vi "Delete SIM Profile.vi"(8 "error in (no error)":errorcluster, 10 "SIM Profile (\"SIM1\")":string="SIM1", 11 "VISA resource name":refnum<visa-resource-name>) -> (0 "error out":errorcluster, 3 "VISA resource name out":refnum<visa-resource-name>)   [LabVIEW 2015, in "Rohde&Schwarz CMXP Base.lvlib"]
doc: "Deletes the SIM profile with the specified name.\n\nAttribute:\nRSCMXPBASE_ATTR_SIM_PROFILE_DELETE\n\nRemote-control command:\nDELete:SIMProfile"
uses:
  <instrlib>/Rohde&Schwarz CMXP Base/Rohde&Schwarz CMXP Base.lvlib
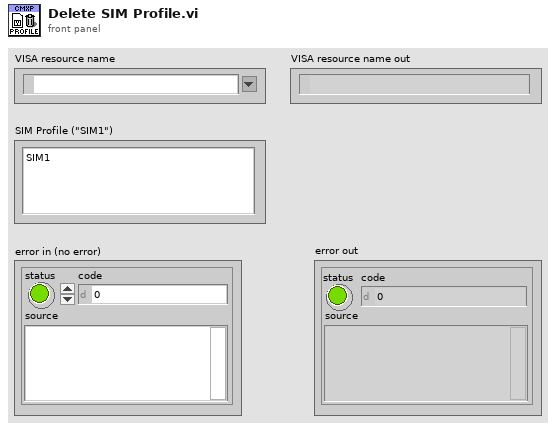
[diagram p1: front panel]
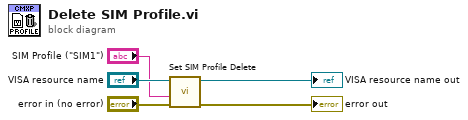
[diagram p0: block diagram]
diagram:
  n1 = call "Set SIM Profile Delete"("error in (no error)"="error in (no error)", "SIM Profile Delete ()"="SIM Profile (\"SIM1\")", "instrument handle"="VISA resource name") -> ("error out"=→"error out":errorcluster, "instrument handle out"=→"VISA resource name out":refnum<visa-resource-name>)  [unwired: 7 in]
